vi "Main.vi"() -> ()   [LabVIEW 2019]
uses:
  <vilib>/myRIO/Common/Instrument Driver Framework/myRIO v1.0/UART/vis/myRIO v1.0 Close UART.vi
  LINE_1.vi
  LINE_2.vi
  <vilib>/myRIO/Common/Instrument Driver Framework/Utilities/vis/FPGA Ref Manager.vi
  <vilib>/myRIO/Common/Instrument Driver Framework/myRIO v1.0/myRIO v1.0 Reset FPGA.vi
  <vilib>/myRIO/Common/Instrument Driver Framework/myRIO v1.0/IRQ/vis/myRIO v1.0 IRQ Info FGV.vi
  <vilib>/myRIO/Common/Instrument Driver Framework/myRIO v1.0/IRQ/vis/myRIO v1.0 Timer IRQ Info FGV.vi
  <vilib>/myRIO/Common/Instrument Driver Framework/myRIO v1.0/IRQ/vis/myRIO v1.0 ISR Agent.vi
  <vilib>/myRIO/Instrument Drivers/Utilities/vis/Reset Index.vi
  <vilib>/myRIO/Common/Instrument Driver Framework/myRIO v1.0/Resource Manager/vis/myRIO v1.0 Block Write Resource Manager.vi
  <vilib>/myRIO/Instrument Drivers/Utilities/Utilities.lvlib
panel:
  in  "error in (no error)":errorcluster
  out "water chart":dbl(graph)
  out "x Chart":dbl(graph)
  out "Sound chart":dbl(graph)
  out "error out 2":errorcluster
  out "LineShow1":string
  out "LineShow2":string
  out "error out":errorcluster
  in  "Stop":bool
  # "[SepperMoter] l1 A/DIO2, l2 A/DIO3, I3 A/DIO4, I5 A/DIO5"
  # "[PIR Sensor]  in A/DIO6, out A/DIO7"
  # "LCD output"
  # "[LED_main] R A/DIO8, G A/DIO9, B A/DIO10"
  # "[Sound Sensor] A/AI0"
  # "[JoyStick]  X A/AI1,  SW A/DIO14"
  # "[LCD] d0 ~ d7   B/DIO0 ~ B/DIO7"
  # "[LCD] E B/DIO8, RW B/DIO9, RS B/DIO10"
  # "[LED_usb]  R B/DIO13, G B/DIO14, B B/DIO15"
  # "[Water Sensor] B/AI1"
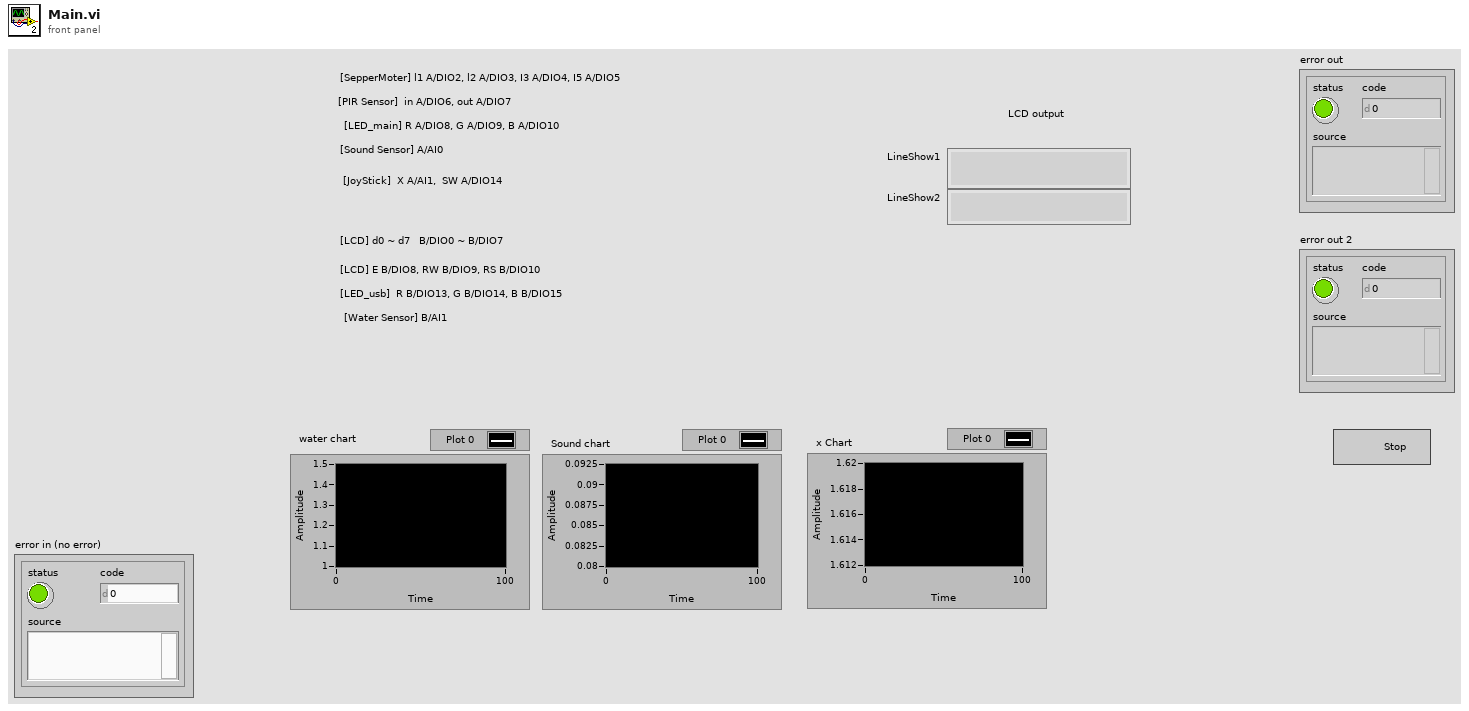
[diagram p1: front panel]
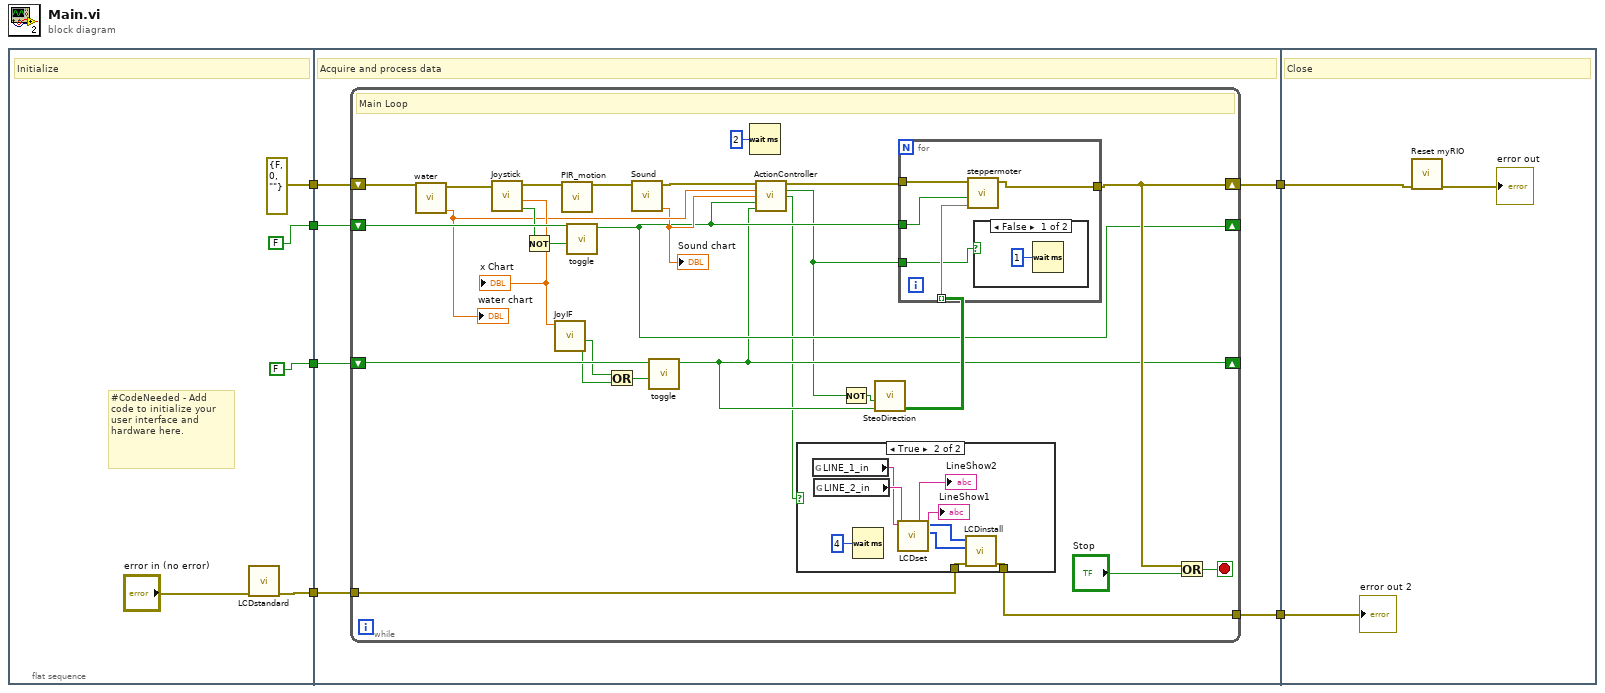
[diagram p0: block diagram]
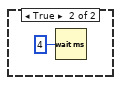
[diagram p3: hidden frame]
diagram:
  n1 = flat-sequence {
    tunnel: [errorcluster {"status"=FALSE, "code"=0, "source"=""} ("error in (no error)")] -> w6
    tunnel: [FALSE ("Boolean 2")] -> w3
    tunnel: [FALSE ("Boolean 2")] -> w2
    tunnel: [w7] -> w1
    tunnel: w6 -> [w17]
    tunnel: [w16] -> w5
    tunnel: [w12] -> w4
    tunnel: w3 -> [w15]
    tunnel: w2 -> [w14]
    tunnel: w1 -> [w13]
    tunnel: w5 -> [w65]
    tunnel: w4 -> [w63]
    frame #0 {
      # "#CodeNeeded - Add code to initialize your user interface and hardware here."
      # "Initialize"
      n2 = call "LCDstandard.vi"("error in (no error)"="error in (no error)") -> ("error out"=w7:errorcluster)  [unwired: 10 in]
    }
    frame #1 {
      # "Acquire and process data"
      n3 = while {
        shift-right: [w41] -> w16
        shift-left: w17 -> [w32]
        shift-right: [w23] -> _
        shift-left: w14 -> [w40]
        shift-right: [w24] -> _
        shift-left: w15 -> [w39]
        tunnel: w13 -> [w20]
        tunnel: [w19] -> w12
        stop <- w44 stop-if-true
        # "Main Loop"
        n4 = call "water.vi"("Error In"=w32) -> ("water Chart"=w26:dbl, "Error Out"=w31:errorcluster)  [unwired: 9 in]
        "water chart" <- w26
        n5 = call "Joystick.vi"("Error In"=w31) -> ("Boolean"=w34:bool, "X Chart"=w38:dbl, "Error Out"=w30:errorcluster)  [unwired: 8 in]
        "x Chart" <- w38
        n6 = Not(x=w34) -> (.not. x?=w33:bool)
        n7 = call "JoyIF.vi"("Numeric"=w38) -> ("down"=w35:bool, "up"=w36:bool)  [unwired: 9 in]
        n8 = call "PIR_motion.vi"("Error In"=w30) -> ("Error Out"=w29:errorcluster)  [unwired: 10 in]
        n9 = call "toggle.vi"("Boolean 3"=w33, "Boolean"=w39) -> ("Boolean 2"=w24:bool)  [unwired: 9 in]
        n10 = Or(x=w36, y=w35) -> (x .or. y?=w37:bool)
        n11 = call "Sound.vi"("Error In"=w29) -> ("Waveform Chart"=w25:dbl, "Error Out"=w28:errorcluster)  [unwired: 9 in]
        "Sound chart" <- w25
        n12 = call "toggle.vi"("Boolean 3"=w37, "Boolean"=w40) -> ("Boolean 2"=w23:bool)  [unwired: 9 in]
        n13 = Wait (ms)(milliseconds to wait=u32 2) -> ()  [unwired: 1 out]
        n14 = call "ActionController.vi"("Error In"=w28, "Water"=w26, "Sound"=w25, "on/off toggle"=w24, "direction toggle 2"=w23) -> ("Error Out"=w27:errorcluster, "감속"=w21:bool, "LCD 변경"=w18:bool)  [unwired: 8 in]
        n15 = case shown="True" w18 {
          tunnel: w20 -> [w46 w51]
          tunnel: [w46 w50] -> w19
          frame False {
          }
          frame True {
            n16 = global read "LINE_1.vi" "LINE_1_in"() -> (w54:string)
            n17 = global read "LINE_2.vi" "LINE_2_in"() -> (w55:string)
            n18 = Wait (ms)(milliseconds to wait=u32 4) -> ()  [unwired: 1 out]
            n19 = call "LCDset.vi"("in in LINE2"=w55, "in LINE1"=w54) -> ("Line1"=→"LineShow1":string, "unsigned byte array"=w49:u8[], "unsigned byte array 2"=w48:u8[], "Line2"=→"LineShow2":string)  [unwired: 6 in]
            n20 = call "LCDinstall.vi"("error in (no error)"=w51, "unsigned byte array"=w49, "unsigned byte array 2"=w48) -> ("error out"=w50:errorcluster)  [unwired: 8 in]
          }
        }
        n21 = Not(x=w21) -> (.not. x?=w22:bool)
        n22 = call "SteoDirection.vi"("방향"=w23, "속도"=w22) -> ("Array"=w42:bool[][])  [unwired: 9 in]
        n23 = for {
          tunnel: w27 -> [w60]
          tunnel: [w58] -> w41
          tunnel: w42 -> [w59] mode=indexing
          tunnel: w24 -> [w57]
          tunnel: w21 -> [w56]
          n24 = call "steppermoter.vi"("Array"=w59, "Boolean"=w57, "Error In"=w60) -> ("Error Out"=w58:errorcluster)  [unwired: 8 in]
          n25 = case shown="False" w56 {
            frame False {
              n26 = Wait (ms)(milliseconds to wait=u32 1) -> ()  [unwired: 1 out]
            }
            frame True {
              n27 = Wait (ms)(milliseconds to wait=u32 4) -> ()  [unwired: 1 out]
            }
          }
        }
        n28 = Or(x=w41, y="Stop") -> (x .or. y?=w44:bool)
      }
    }
    frame #2 {
      # "Close"
      n29 = call <vilib>:"Reset myRIO.vi"("error in (no error)"=w65) -> ("error out"=→"error out":errorcluster)  [unwired: 10 in]
      "error out 2" <- w63
    }
  }
